vi "Write Tags.vi"(8 "error in (no error)":errorcluster, 11 "State in":T1={"State"=enum."Idle", "Start Time"=timestamp(0 s since 1904-01-01), "Configuration"={"Cycle Period"=0.0, "PID 2 Parameters"={"Input Device"=enum."4-20mA", "Output Device"=enum."Default", "Setpoint"=0.0, "PID gains"={"proportional gain (Kc)"=0.0, "integral time (Ti, min)"=0.0, "derivative time (Td, min)"=100.0}, "output range"={"output low"=0.0, "output high"=1.0}}, "Manual Entry"=0.0, "Auto?"=TRUE, "4-20mA Input Settings"={"Input Channel "=0}, "4-20mA Out Settings"={"Output DAQ Task"=""}, "Input Channel Tag Name "=""}, "Current Time"=timestamp(0 s since 1904-01-01), "PID 1 Parameters"={"Setpoint"=0.0, "PID gains"={"proportional gain (Kc)"=1.0, "integral time (Ti, min)"=0.01, "derivative time (Td, min)"=0.0}}, "First Iteration"=FALSE, "Data"={"4-20mA Input"=0.0, "PID 2 Process Variable"=0.0, "PID 2 Output"=0.0, "4-20mA Output"=0.0}, "Process Name"="", "Pump On?"=enum."Off", "Input Error"=FALSE, "Output Error"=FALSE, "Log Started"=FALSE, "Current Setpoint"=0.0} {"Configuration"."PID 2 Parameters"."output range"."output low" format="%.2f"; "Configuration"."PID 2 Parameters"."output range"."output high" min=0.0 max=100.0 format="%.2f"; "Configuration"."PID 2 Parameters"."PID gains"."derivative time (Td, min)" format="%.3f"; "Configuration"."PID 2 Parameters"."PID gains"."integral time (Ti, min)" format="%.3f"; "Configuration"."PID 2 Parameters"."PID gains"."proportional gain (Kc)" format="%.3f"; "PID 1 Parameters"."PID gains"."derivative time (Td, min)" format="%.3f"; "PID 1 Parameters"."PID gains"."integral time (Ti, min)" format="%.3f"; "PID 1 Parameters"."PID gains"."proportional gain (Kc)" format="%.3f"}) -> (0 "error out":errorcluster, 3 "State out":T1={"State"=enum."Idle", "Start Time"=timestamp(0 s since 1904-01-01), "Configuration"={"Cycle Period"=0.0, "PID 2 Parameters"={"Input Device"=enum."4-20mA", "Output Device"=enum."Default", "Setpoint"=0.0, "PID gains"={"proportional gain (Kc)"=0.0, "integral time (Ti, min)"=0.0, "derivative time (Td, min)"=100.0}, "output range"={"output low"=0.0, "output high"=1.0}}, "Manual Entry"=0.0, "Auto?"=TRUE, "4-20mA Input Settings"={"Input Channel "=0}, "4-20mA Out Settings"={"Output DAQ Task"=""}, "Input Channel Tag Name "=""}, "Current Time"=timestamp(0 s since 1904-01-01), "PID 1 Parameters"={"Setpoint"=0.0, "PID gains"={"proportional gain (Kc)"=1.0, "integral time (Ti, min)"=0.01, "derivative time (Td, min)"=0.0}}, "First Iteration"=FALSE, "Data"={"4-20mA Input"=0.0, "PID 2 Process Variable"=0.0, "PID 2 Output"=0.0, "4-20mA Output"=0.0}, "Process Name"="", "Pump On?"=enum."Off", "Input Error"=FALSE, "Output Error"=FALSE, "Log Started"=FALSE, "Current Setpoint"=0.0} {"Configuration"."PID 2 Parameters"."output range"."output low" format="%.2f"; "Configuration"."PID 2 Parameters"."output range"."output high" min=0.0 max=100.0 format="%.2f"; "Configuration"."PID 2 Parameters"."PID gains"."derivative time (Td, min)" format="%.3f"; "Configuration"."PID 2 Parameters"."PID gains"."integral time (Ti, min)" format="%.3f"; "Configuration"."PID 2 Parameters"."PID gains"."proportional gain (Kc)" format="%.3f"; "PID 1 Parameters"."PID gains"."derivative time (Td, min)" format="%.3f"; "PID 1 Parameters"."PID gains"."integral time (Ti, min)" format="%.3f"; "PID 1 Parameters"."PID gains"."proportional gain (Kc)" format="%.3f"})   [LabVIEW 2018, in "4-20mA Module.lvlib" / "4-20mA Module Engine.lvlib"]
uses:
  4-20mA Module Engine.lvlib
  State Cluster.ctl
  State Enum.ctl
  Pressure Transmitter/Pressure Transmitter Device Settings.ctl
  Pressure Reg Module/Pressure Regulator Device Settings.ctl
  Measure Instrument/PID 1 Parameters Cluster.ctl
  Tag VIs/Tag FGV Operation Enum.ctl
  Shared Variables/Dynamic Shared Variables.lvlib
  Pressure Transmitter/Pressure Transmitter Library.lvlib
  Pressure Reg Module/Pressure Regulator Library.lvlib
panel:
  # "Instrument Settings"
  # "Instrument Settings"
  # "Instrument Settings"
  # "Instrument Settings"
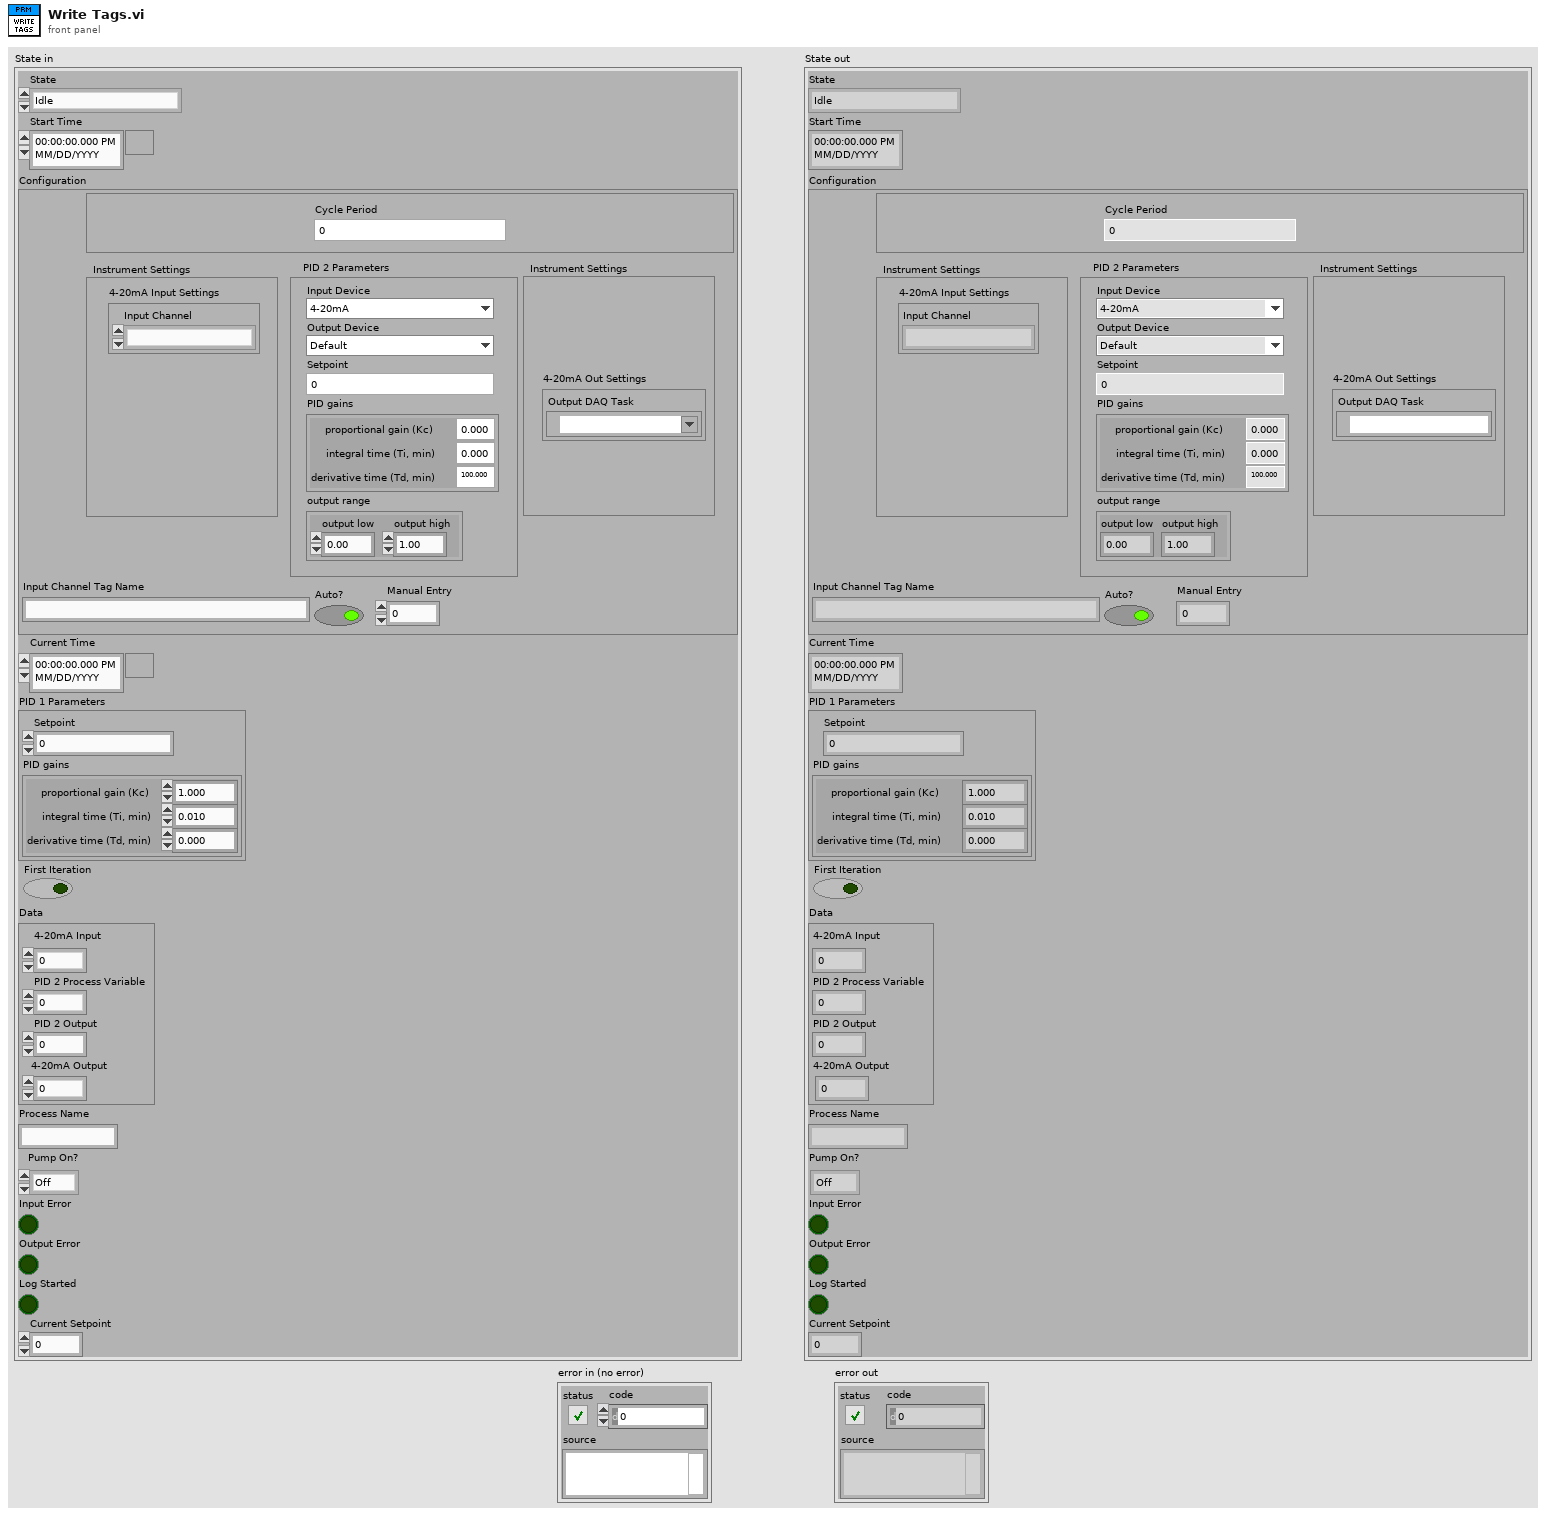
[diagram p1: front panel]
types:
  T1 = typedef "4-20mA Module.lvlib/4-20mA Module Engine.lvlib/State Cluster.ctl" = cluster{"State":T2, "Start Time":timestamp, "Configuration":cluster{"Cycle Period":dbl, "PID 2 Parameters":cluster{"Input Device":enum16{"Default", "4-20mA"}, "Output Device":enum16{"Default", "Equilibar Pressure Reg", "Flow Regulator"}, "Setpoint":dbl, "PID gains":cluster{"proportional gain (Kc)":dbl, "integral time (Ti, min)":dbl, "derivative time (Td, min)":dbl}, "output range":cluster{"output low":dbl, "output high":dbl}}, "Manual Entry":dbl, "Auto?":bool, "4-20mA Input Settings":T3, "4-20mA Out Settings":T4, "Input Channel Tag Name ":string}, "Current Time":timestamp, "PID 1 Parameters":T5, "First Iteration":bool, "Data":cluster{"4-20mA Input":dbl, "PID 2 Process Variable":dbl, "PID 2 Output":dbl, "4-20mA Output":dbl}, "Process Name":string, "Pump On?":enum16{"Off", "On", "Not Initialized"}, "Input Error":bool, "Output Error":bool, "Log Started":bool, "Current Setpoint":dbl}
  T2 = typedef "4-20mA Module.lvlib/4-20mA Module Engine.lvlib/State Enum.ctl" = enum16{"Measuring", "Idle", "Paused"}
  T3 = typedef "Pressure Transmitter Library.lvlib/Pressure Transmitter Device Settings.ctl" = cluster{"Input Channel ":u16}
  T4 = typedef "Pressure Regulator Library.lvlib/Pressure Regulator Device Settings.ctl" = cluster{"Output DAQ Task":refnum<k21>}
  T5 = typedef "PID 1 Parameters Cluster.ctl" = cluster{"Setpoint":dbl, "PID gains":cluster{"proportional gain (Kc)":dbl, "integral time (Ti, min)":dbl, "derivative time (Td, min)":dbl}}
  T6 = typedef "Tag FGV Operation Enum.ctl" = enum16{"Init", "Set Notification Queue", "Create Tag", "Commit", "Write Tag (Numeric)", "Write Tag (Boolean)", "Read All Tags", "Read One Tag", "Delete Tag Category", "Set Alarm Parameters (Numeric)", "Set Alarm Parameters (Boolean)", "Enable All Alarms", "Disable All Alarms", "Delete All Tags", "Read Alarms", "Ack Alarm", "Read Alarm Parameters (Numeric)", "Read Alarm Parameters (Boolean)"}
  T7 = typedef "4-20mA Module.lvlib/4-20mA Module Tag Names Cluster.ctl" = cluster{"4-20mA Input":string, "PID 2 Out Tag":string, "4-20mA Output":string, "Input Device Tag":string, "Output Device Tag":string}
  T8 = cluster{"4-20mA Input":dbl, "PID 2 Process Variable":dbl, "PID 2 Output":dbl, "4-20mA Output":dbl}
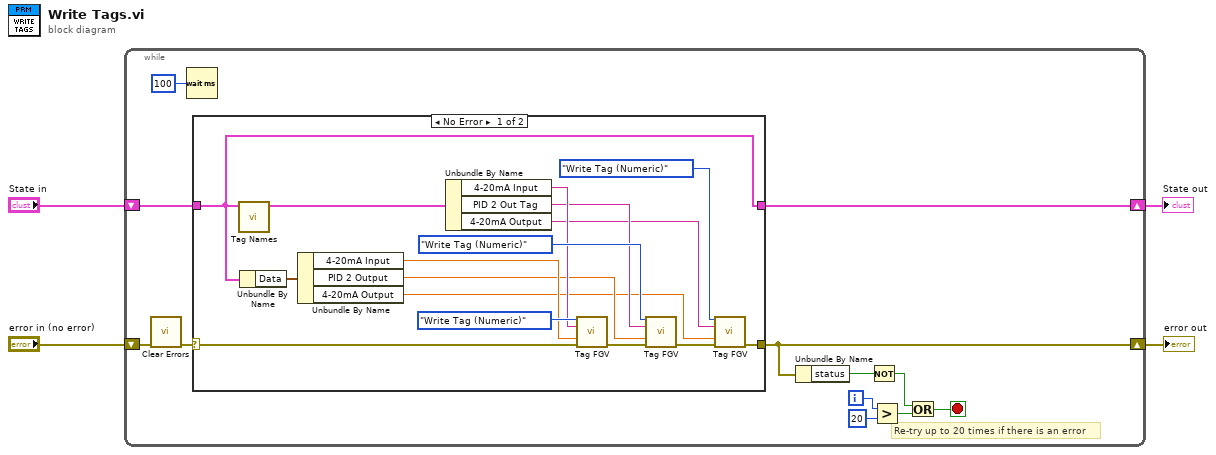
[diagram p0: block diagram]
diagram:
  n1 = while {
    shift-right: [w10] -> w3
    shift-left: "error in (no error)" -> [w8]
    shift-right: [w15] -> w1
    shift-left: "State in" -> [w16]
    i -> [w6]
    stop <- w14 stop-if-true
    # "Re-try up to 20 times if there is an error"
    n2 = call <vilib>:"Clear Errors.vi"("error in (no error)"=w8) -> ("error out"=w7:errorcluster)  [unwired: 5 in, 1 out]
    n3 = Wait (ms)(milliseconds to wait=u32 100) -> ()  [unwired: 1 out]
    n4 = case shown="No Error" w7 {
      selector: w7 -> [w32 w34]
      tunnel: [w17 w34] -> w10
      tunnel: w16 -> [w23 w33]
      tunnel: [w23 w33] -> w15
      frame No Error {
        n5 = call "Tag Names.vi"("State in"=w23) -> ("4-20mA Module Tag Names"=w27:T7)  [unwired: 8 in, 2 out]
        n6 = Unbundle By Name(w23) -> ("Data"=w21:T8)
        n7 = Unbundle By Name(w21) -> ("4-20mA Input"=w20:dbl, "PID 2 Output"=w19:dbl, "4-20mA Output"=w18:dbl)
        n8 = Unbundle By Name(w27) -> ("4-20mA Input"=w26:string, "PID 2 Out Tag"=w25:string, "4-20mA Output"=w24:string)
        n9 = call "Tag FGV.vi"("Operation"=Tag_FGV_Operation_Enum."Write Tag (Numeric)", "Tag Name"=w26, "Data"=w20, "error in (no error)"=w32) -> ("error out"=w29:errorcluster)  [unwired: 4 in, 7 out]
        n10 = call "Tag FGV.vi"("Operation"=Tag_FGV_Operation_Enum."Write Tag (Numeric)", "Tag Name"=w25, "Data"=w19, "error in (no error)"=w29) -> ("error out"=w28:errorcluster)  [unwired: 4 in, 7 out]
        n11 = call "Tag FGV.vi"("Operation"=Tag_FGV_Operation_Enum."Write Tag (Numeric)", "Tag Name"=w24, "Data"=w18, "error in (no error)"=w28) -> ("error out"=w17:errorcluster)  [unwired: 4 in, 7 out]
      }
      frame Error {
      }
    }
    n12 = Unbundle By Name(w10) -> ("status"=w9:bool)
    n13 = Not(x=w9) -> (.not. x?=w13:bool)
    n14 = Greater?(x=w6, y=20) -> (0:w11:bool)
    n15 = Or(x=w13, y=w11) -> (x .or. y?=w14:bool)
  }
  "error out" <- w3
  "State out" <- w1
